vi "Untitled 2.vi"() -> ()   [LabVIEW 2017, in "labview-standard-library.lvlib"]
uses:
  labview-standard-library.lvlib
  universial-controls/Driver_inputs.ctl
panel:
  out "Waveform Graph":dbl[](graph)
  out "error out":errorcluster
  in  "error in (no error)":errorcluster
  out "notifier out":refnum<notifier>
  in  "notifier in":refnum<notifier>
  in  "Driver controls in":T1
  out "Driver controls out":T1
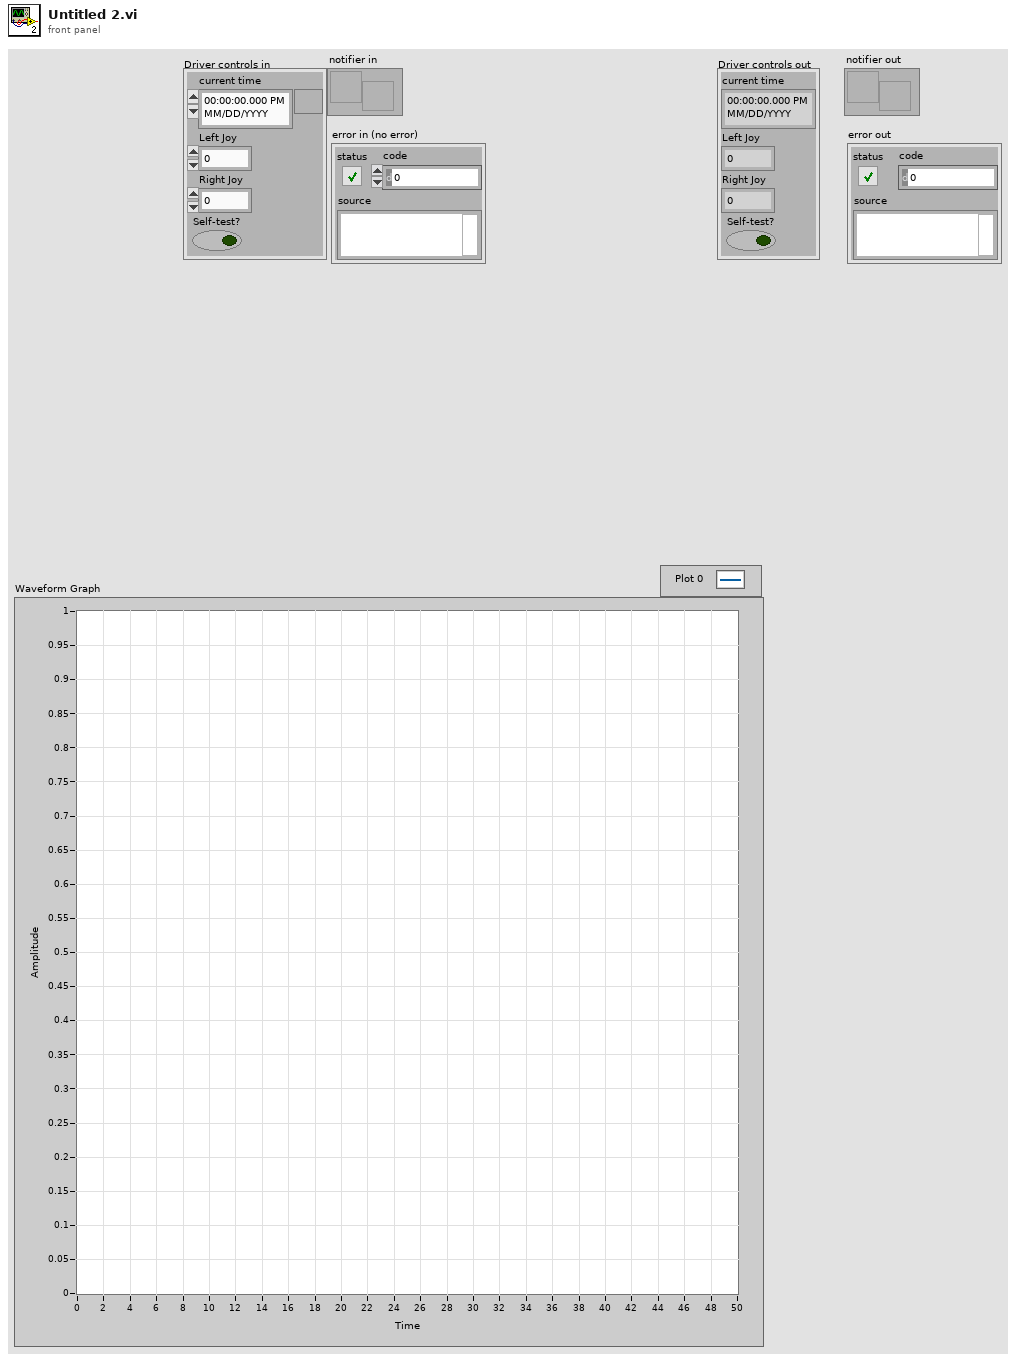
[diagram p1: front panel]
types:
  T1 = typedef "labview-standard-library.lvlib/Driver_inputs.ctl" = cluster{"current time":timestamp, "Left Joy":dbl, "Right Joy":dbl, "Self-test?":bool}
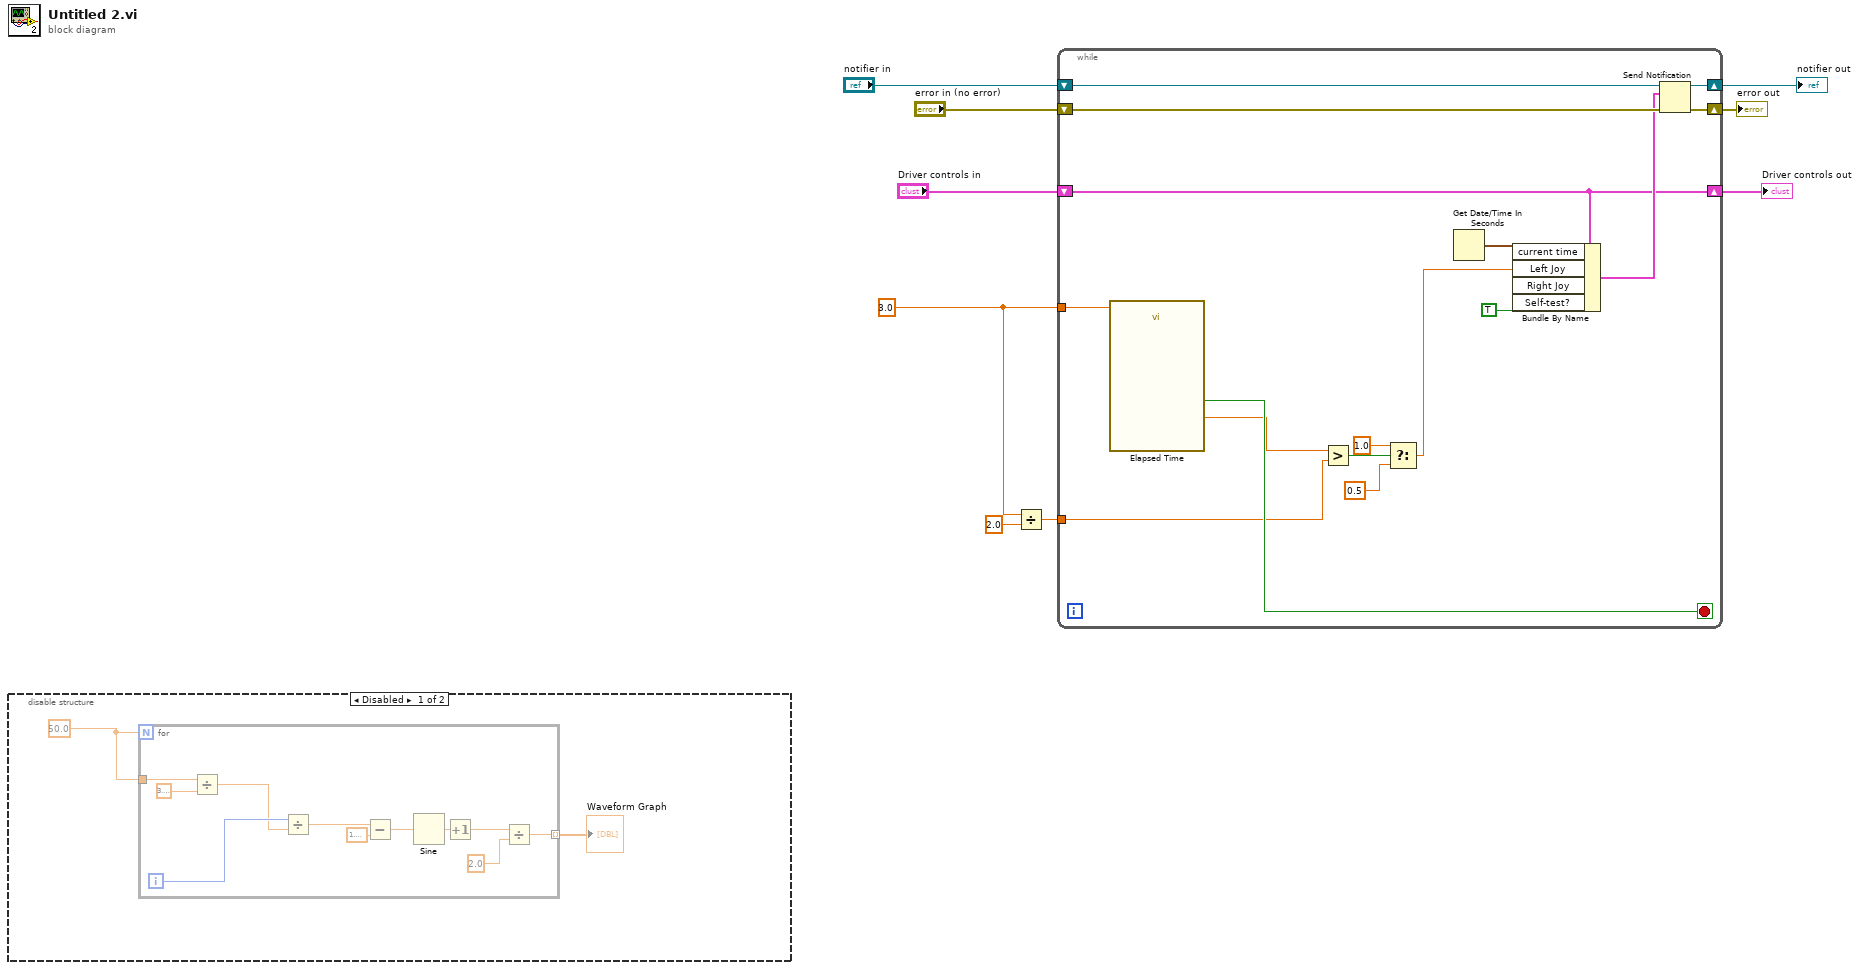
[diagram p0: block diagram]
diagram:
  w3 = 3.0 ("Time Target (s)")
  n1 = disable-structure shown="Disabled" {
    frame Disabled {
      w10 = 50.0 ("x")
      n2 = for {
        N: w10 -> [_]
        tunnel: [w12] -> w11 mode=indexing
        tunnel: w10 -> [w17]
        i -> [w22]
        n3 = Divide(x=w17, y=3.141592653589793) -> (x/y=w16:dbl)
        n4 = Divide(x=w22, y=w16) -> (x/y=w20:dbl)
        n5 = Subtract(x=w20, y=1.5707963267948966) -> (x-y=w21:dbl)
        n6 = Sine(x=w21) -> (sin(x)=w14:dbl)
        n7 = Increment(x=w14) -> (x+1=w13:dbl)
        n8 = Divide(x=w13, y=2.0) -> (x/y=w12:dbl)
      }
      "Waveform Graph" <- w11
    }
    frame Enabled {
    }
  }
  n9 = Divide(x=w3, y=2.0) -> (x/y=w2:dbl)
  n10 = while {
    shift-right: [w35] -> w8
    shift-left: "notifier in" -> [w36]
    shift-right: [w33] -> w6
    shift-left: "error in (no error)" -> [w34]
    shift-right: [w31] -> w4
    shift-left: "Driver controls in" -> [w31]
    tunnel: w3 -> [w28]
    tunnel: w2 -> [w27]
    stop <- w30 stop-if-true
    n11 = call "Elapsed Time"("Time Target (s)"=w28) -> ("Elapsed Time (s)"=w26:dbl, "Time has Elapsed"=w30:bool)  [unwired: 11 in, 6 out]
    n12 = Greater?(x=w26, y=w27) -> (0:w29:bool)
    n13 = Select(t=1.0, s=w29, f=0.5) -> (s? t:f=w23:dbl)
    n14 = Get Date/Time In Seconds() -> (seconds since 1Jan1904=w37:timestamp)
    n15 = Bundle By Name(cluster=w31, "current time"=w37, "Left Joy"=w23, "Self-test?"=TRUE) -> (w32:T1)  [unwired: 1 in]
    n16 = Send Notification(notification=w32, notifier=w36, error in (no error)=w34) -> (notifier out=w35:refnum<notifier>, error out=w33:errorcluster)
  }
  "Driver controls out" <- w4
  "notifier out" <- w8
  "error out" <- w6
